vi "Get Subscriptions.vi"(8 "error in (no error)":errorcluster, 11 "Data Tracker Msg in":refnum<class "Data Tracker Msg.lvclass">) -> (0 "error out":errorcluster, 2 "Subscriptions":refnum<class "Data.lvclass">[](array[class]), 3 "Data Tracker Msg out":refnum<class "Data Tracker Msg.lvclass">)   [LabVIEW 2020, in "Data Tracker.lvlib" / "Data Tracker Msg.lvclass"]
doc: "Return the subscriptions associated with the instance of the Data Tracker Msg."
uses:
  Data Tracker Msg.lvclass
  PPL/HDH.Data.Generic.lvlibp/Data.lvclass
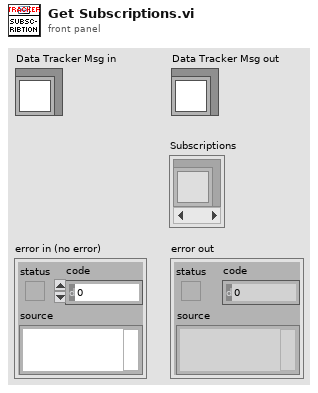
[diagram p1: front panel]
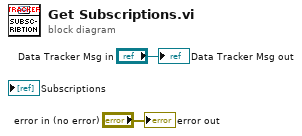
[diagram p0: block diagram]
diagram:
  "error out" <- "error in (no error)"
  "Data Tracker Msg out" <- "Data Tracker Msg in"
